vi "BPS Driver.vi"(8 "Scaling Factor":fxp<+,27,10>, 9 "Offset":fxp<+/-,26,5>, 11 "Signal In":fxp<+/-,26,5>) -> (2 "Brake Pressure (psi)":fxp<+/-,27,16>, 3 "Sensor OK?":bool)   [LabVIEW 2014]
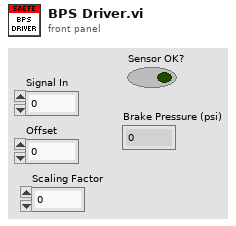
[diagram p1: front panel]
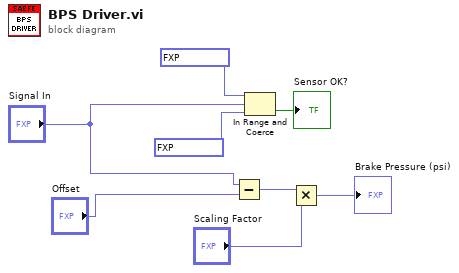
[diagram p0: block diagram]
diagram:
  n1 = Subtract(x="Signal In", y="Offset") -> (x-y=w7:fxp<+/-,27,6>)
  n2 = In Range and Coerce(upper limit=fxp<+/-,14,5> 4.599609375, x="Signal In", lower limit=fxp<+/-,14,5> 0.400390625) -> (In Range?=→"Sensor OK?":bool)  [unwired: 1 out]
  n3 = Multiply(x=w7, y="Scaling Factor") -> (x*y=→"Brake Pressure (psi)":fxp<+/-,27,16>)
